vi "Robot Global Data.vi"() -> ()   [LabVIEW 2017]
doc: "This global VI can contain as many global variables as you need. Place a control on the panel, give it a good name. To read or write to it from a VI, drag the icon to the diagram of that VI. You can also drag from the project. Click on the node to change which global you access. You shouldn't have multiple locations writing to a global or it will cause a race-condition."
uses:
  <vilib>/Rock Robotics/WPI/Camera/WPI_CameraImageSize.ctl
  <vilib>/Rock Robotics/WPI/DriverStation/WPI_DriverStationRobotMode2.ctl
panel:
  in  "Lift Encoder Offset":dbl=-3166.0
  in  "Teleop Enabled":bool
  in  "Carrage Slow Eject":dbl=0.5
  in  "Auto Current Based Move (C)":dbl
  in  "Auto Start Angle (B)":dbl
  in  "Auto Turn Complete":bool
  in  "Auto Array":string[](array[string])
  in  "Auto Code":string
  in  "Take Slack Speed":dbl
  in  "Adjust Position Speed":dbl
  in  "Adjusted Position Offset":dbl
  in  "PreAdjust Position Offset":dbl
  in  "Adjusted Position":dbl
  in  "PreAdjust Position":dbl
  in  "Reset Lift at Intake Position":bool
  in  "Lift Decent Speed for Climb":dbl=-0.1
  in  "Invert Manual Lift":bool
  in  "Climb Hook Status":bool
  in  "Reset Position":dbl
  in  "Reset Position Offset":dbl=16280.0
  in  "Hold Hook Angle":i32=90
  in  "Deploy Hook Angle":i32=180
  in  "Hold Angle R":i32=100
  in  "Hold Angle L":i32
  in  "Release Angle R":i32=30
  in  "Release Angle L":i32=180
  in  "Auto Move Done":bool
  in  "Auto Turn Before Drive Threshold":dbl=30.0
  in  "Lift Reference Point":dbl
  in  "Intake Position Offset":dbl=-1657.0
  in  "Climb Position Offset":dbl=111350.0
  in  "Climb Position":dbl
  in  "Scale Position High Offset":dbl=127815.0
  in  "Scale Position Mid Offset":dbl=110364.0
  in  "Scale Position Low Offset":dbl=89679.0
  in  "Switch Position Offset":dbl=45683.0
  in  "Cube Hold Position Offset":dbl=11812.0
  in  "Intake Wheel Intake Speed":dbl=0.75
  in  "Carrage Eject":dbl=1.0
  in  "Carrage Intake":dbl=-0.5
  in  "Saved Lift Position":dbl
  in  "Auto Lift Command (L)":dbl
  in  "Auto Orientation Angle (A)":dbl
  in  "Auto Distance (M)":dbl
  in  "Auto Movement Angle (T)":dbl
  in  "Warning":bool
  in  "Estop":bool
  in  "Blink":bool
  out "Teleop Elapsed":dbl
  in  "Reset Encoder":bool
  in  "FR Encoder":dbl
  in  "Current Lift Position":dbl
  in  "Ramp Tail Status":bool=TRUE
  in  "Intake Short Status":bool
  in  "Intake Long Status":bool
  in  "Cycle Pause":dbl=1.0
  in  "Cycle Timeout":dbl=2.0
  in  "Intake Secure":bool
  in  "Intake Seen":bool
  in  "Scale Position High":dbl
  in  "Scale Position Mid":dbl
  in  "Scale Position Low":dbl
  in  "Switch Position":dbl
  in  "Cube Hold Position":dbl
  in  "Intake Position":dbl
  in  "Zero Gyro":bool
  in  "Toggle Field Orient":bool=TRUE
  in  "Swrv Spin Zeros":path=path "/home/lvuser/spinzeros.csv"
  in  "First Enabled Loop":bool
  in  "BR Zero":dbl
  in  "BL Zero":dbl
  in  "FR Zero":dbl
  in  "FL Zero":dbl
  in  "Gyro":dbl
  in  "Robot Mode":T1
  in  "image size":T2=enum."320x240"
  in  "Enable Vision":bool
  # "Process Variables that are written to in Periodic\n\nThese are the actual sent setpoints based on the\noffsets from the reference point"
  # "Off - Tail Out\nOn - Tail Up"
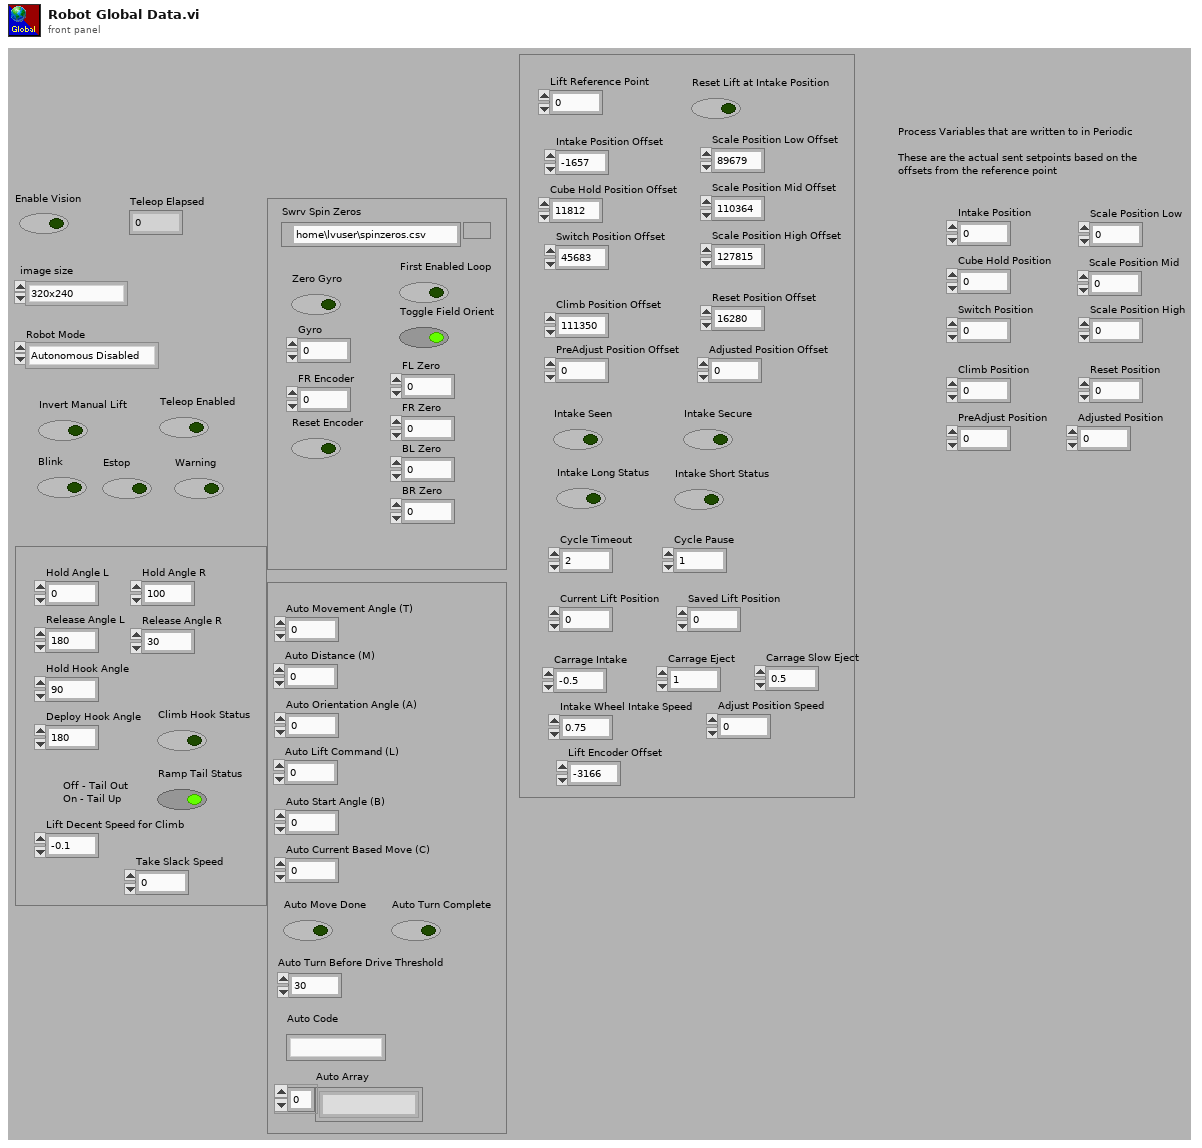
[diagram p1: front panel]
types:
  T1 = typedef "WPI_DriverStationRobotMode2.ctl" = enum16{"Autonomous Disabled", "Autonomous Enabled", "Teleop Disabled", "Teleop Enabled", "Disconnected", "Finish", "Test Disabled", "Test Enabled", "Emergency Stopped"}
  T2 = typedef "WPI_CameraImageSize.ctl" = enum16{"640x480", "320x240", "160x120", "Custom"}
diagram:
